vi "RS_FSP.vi"(4 "error in":T13, 7 "Command":string) -> (0 "error out":T13, 3 "Response":T11)   [LabVIEW 2018]
uses:
  MOKO_LabViewLibrary/MokoLowLevel/MokoLowLovelControl/MLLC_Error.ctl
  MOKO_LabViewLibrary/MokoLowLevel/MokoLowLovelControl/MLLC_Mode.ctl
  MOKO_LabViewLibrary/MokoLowLevel/MokoLowLovelControl/MLLC_Response.ctl
  MOKO_LabViewLibrary/MokoLowLevel/MokoLowLovelControl/MLLC_ConnectCluster.ctl
  MOKO_LabViewLibrary/MokoLowLevel/MokoLowLovelControl/MLLC_InterfaceType.ctl
  MOKO_LabViewLibrary/MokoLowLevel/MokoLowLovelControl/MLLC_OpenedSession.ctl
  MOKO_LabViewLibrary/MokoLowLevel/MokoLowLovelControl/MLLC_InterfaceSettings.ctl
  MOKO_LabViewLibrary/MokoLowLevel/MokoLowLovelControl/MLLC_InterfaceKind.ctl
  MOKO_LabViewLibrary/MokoLowLevel/MokoLowLovelControl/MLLC_DriverName.ctl
  MOKO_LabViewLibrary/MokoLowLevel/MokoLowLovelControl/MLLC_ErrorCode.ctl
  MOKO_LabViewLibrary/MokoLowLevel/MokoLowLovelControl/MLLC_ResponseInit.ctl
  MOKO_LabViewLibrary/MokoLowLevel/MokoLowLovelControl/MLLC_Request.ctl
  MOKO_LabViewLibrary/MokoLowLevel/MokoLowLovelControl/MLLC_Delay.ctl
panel:
  in  "Request":T1="*IDN?"
  in  "Response Init":T2="Rohde&Schwarz,FSP-30"
  in  "Error Code":T3=5450
  in  "Driver Name":T4="RS_FSP"
  in  "Settings":T10={"Saved Data"=variant, "Data"={"Connect"={"InterfaceType"=enum."VISA", "OpenedSession"="TCPIP0::169.254.1.110::inst0::INSTR", "InterfaceSettings"={"Interface"=enum."Ethernet", "EOS 4 read"=enum."LF (\\n)", "EOS 4 write"=enum."LF (\\n)", "TMO, ms"=10000, "Sett"=variant}}}}
  in  "Mode":T12=enum."Check"
  # "RS_FSP"
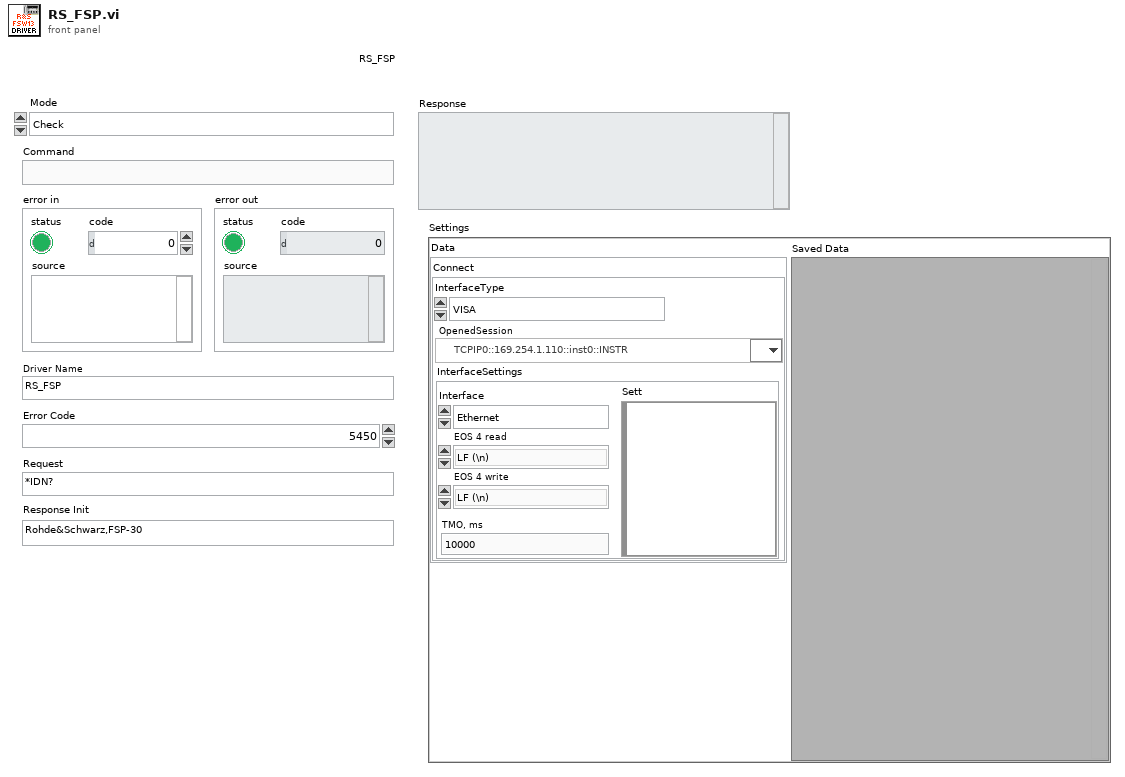
[diagram p1: front panel]
types:
  T1 = typedef "MLLC_Request.ctl" = string
  T2 = typedef "MLLC_ResponseInit.ctl" = string
  T3 = typedef "MLLC_ErrorCode.ctl" = u32
  T4 = typedef "MLLC_DriverName.ctl" = string
  T5 = typedef "MLLC_ConnectCluster.ctl" = cluster{"InterfaceType":T6, "OpenedSession":T7, "InterfaceSettings":T8}
  T6 = typedef "MLLC_InterfaceType.ctl" = enum16{"VISA", "Prologix USB-GPIB"}
  T7 = typedef "MLLC_OpenedSession.ctl" = refnum<visa-resource-name>
  T8 = typedef "MLLC_InterfaceSettings.ctl" = cluster{"Interface":T9, "EOS 4 read":enum16{"Default (=EOS 4 write)", "CR (\\r)", "LF (\\n)", "None"}, "EOS 4 write":enum16{"CR+LF (\\r\\n)", "CR (\\r)", "LF (\\n)", "None"}, "TMO, ms":i32, "Sett":variant}
  T9 = typedef "MLLC_InterfaceKind.ctl" = enum16{"RS232", "GPIB", "USB", "Ethernet", "another"}
  T10 = cluster{"Saved Data":variant, "Data":cluster{"Connect":T5}}
  T11 = typedef "MLLC_Response.ctl" = string
  T12 = typedef "MLLC_Mode.ctl" = enum16{"get", "set", "close", "Init", "Check"}
  T13 = typedef "MLLC_Error.ctl" = errorcluster
  T14 = typedef "MLLC_Delay.ctl" = dbl
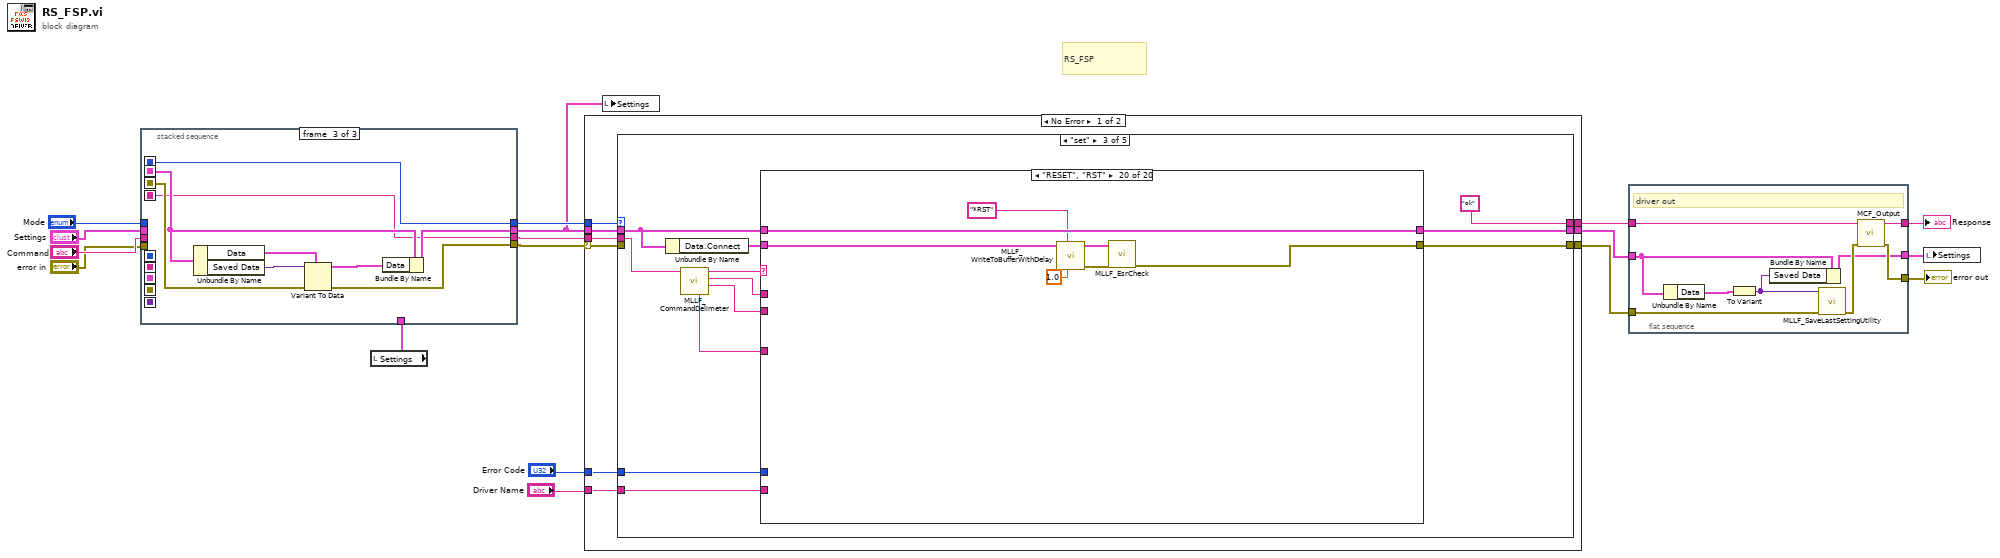
[diagram p0: block diagram]
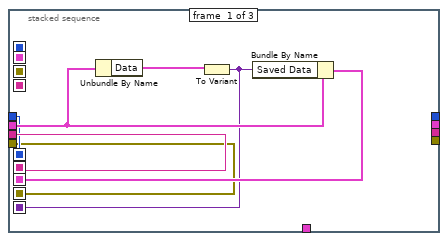
[diagram p2: hidden frame]
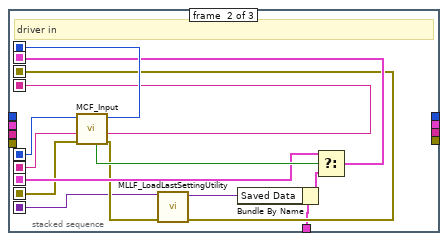
[diagram p3: hidden frame]
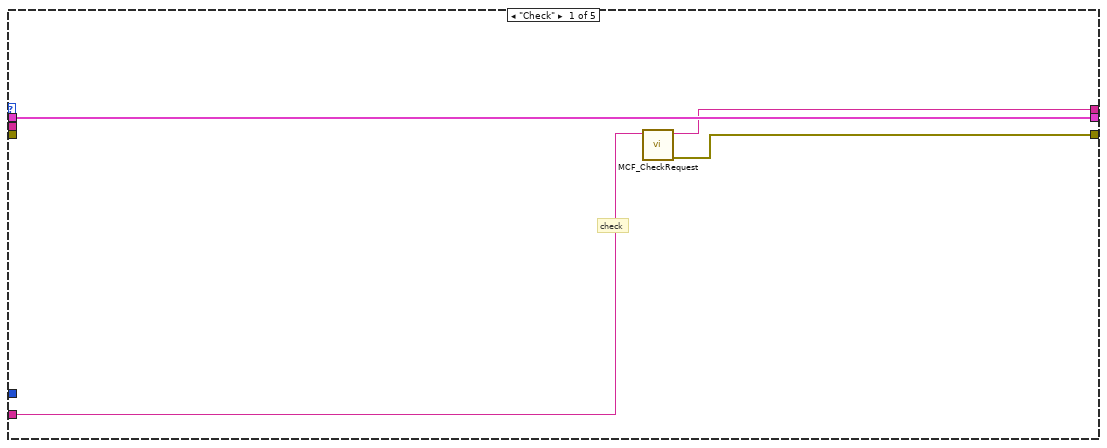
[diagram p4: hidden frame]
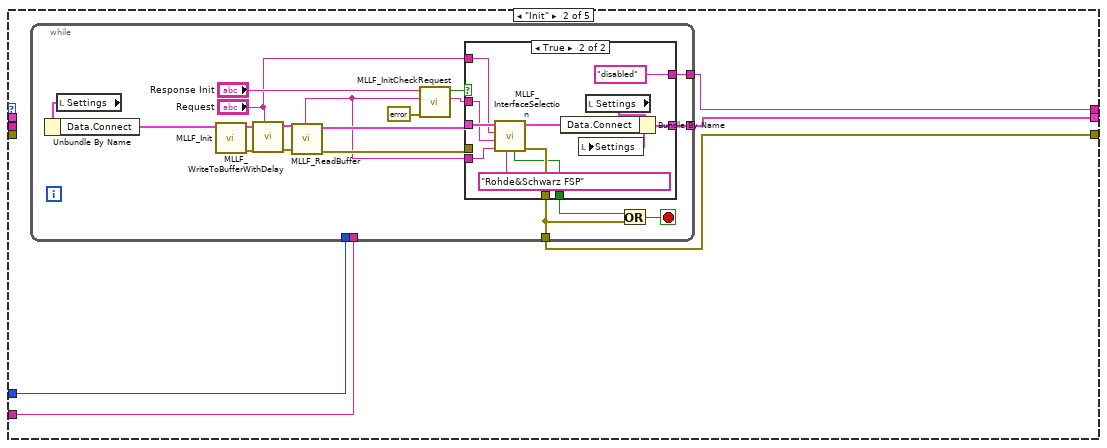
[diagram p5: hidden frame]
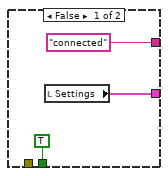
[diagram p6: hidden frame]
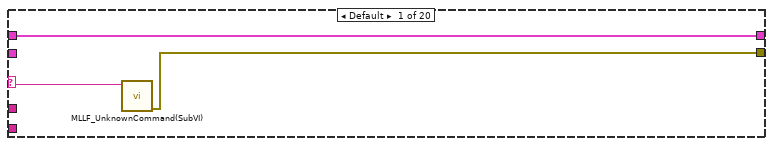
[diagram p7: hidden frame]
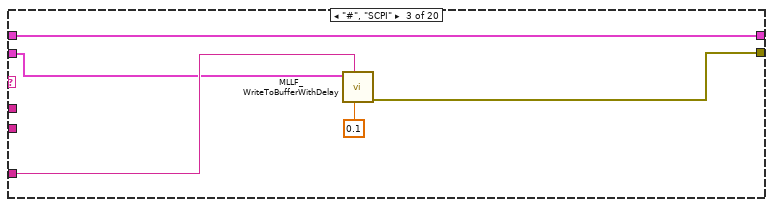
[diagram p9: hidden frame]
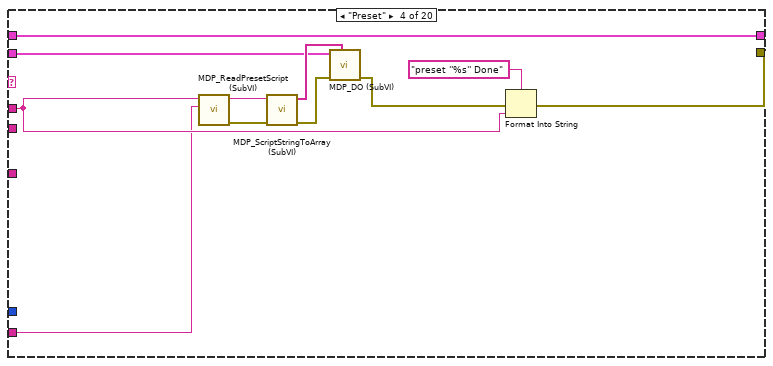
[diagram p10: hidden frame]
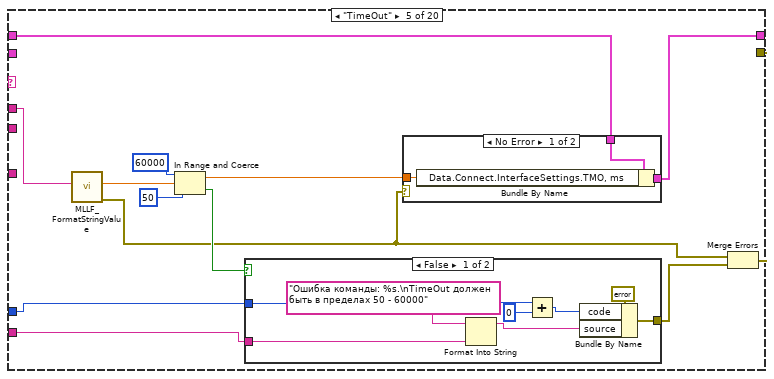
[diagram p11: hidden frame]
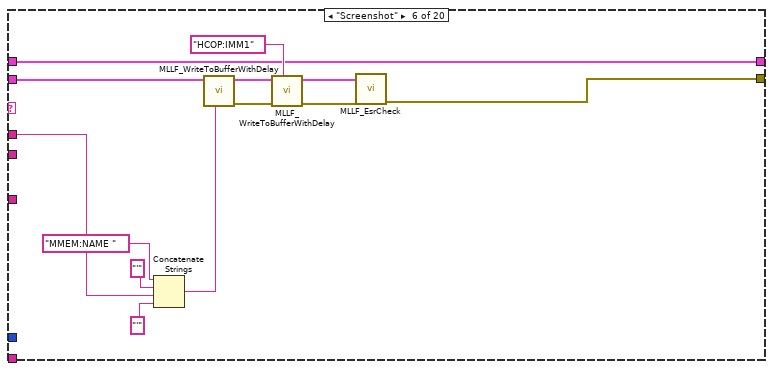
[diagram p14: hidden frame]
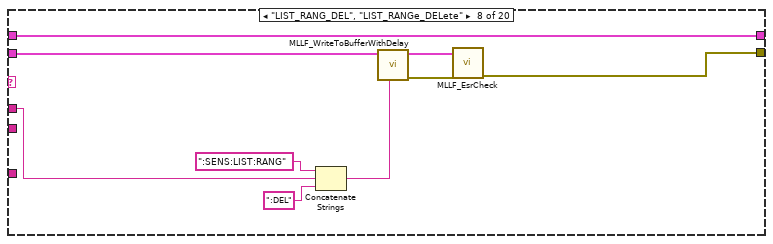
[diagram p16: hidden frame]
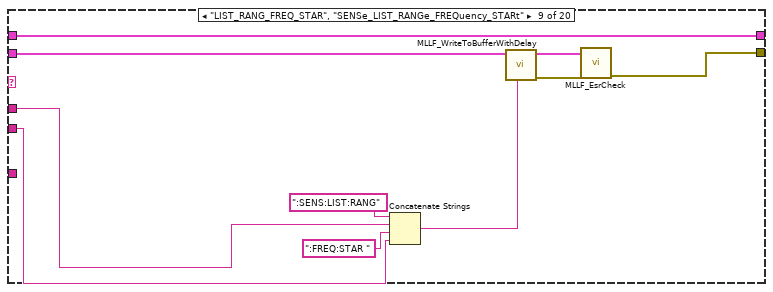
[diagram p17: hidden frame]
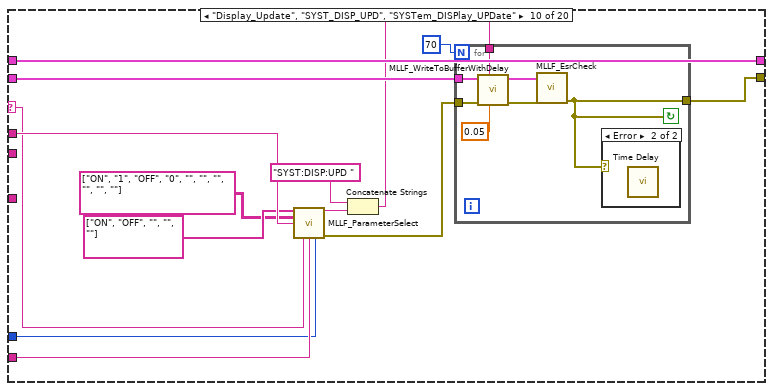
[diagram p18: hidden frame]
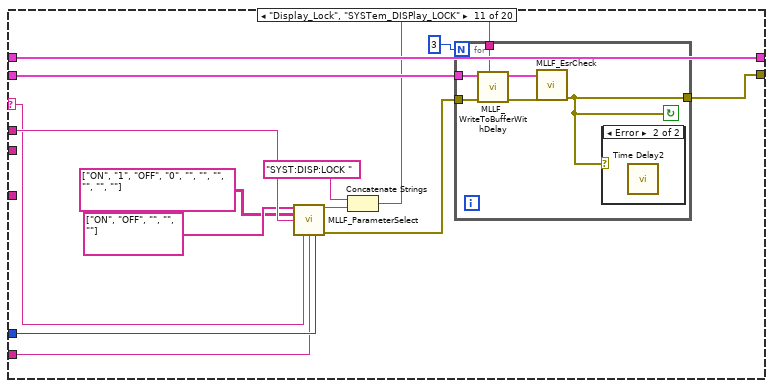
[diagram p20: hidden frame]
diagram:
  # "RS_FSP"
  n1 = local read "Settings"() -> (w15:T10)
  n2 = stacked-sequence {
    seq-local: [w20 _ _] -> [_ w36 _]
    seq-local: [w19 _ _] -> [_ w37 _]
    seq-local: [w22 _ _] -> [_ w32 _]
    seq-local: [w18 _ _] -> [_ w31 _]
    seq-local: [w21 _ _] -> [_ w27 _]
    seq-local: [_ w28 _] -> [_ _ w44]
    seq-local: [_ w38 _] -> [_ _ w41]
    seq-local: [_ w35 _] -> [_ _ w40]
    seq-local: [_ w34 _] -> [_ _ w45]
    tunnel: "Command" -> [w20 _ _]
    tunnel: "Mode" -> [w19 _ _]
    tunnel: "error in" -> [w18 _ _]
    tunnel: "Settings" -> [w23 _ _]
    tunnel: w15 -> [_ w26 _]
    tunnel: [_ _ w40] -> w8
    tunnel: [_ _ w43] -> w9
    tunnel: [_ _ w42] -> w7
    tunnel: [_ _ w41] -> w10
    frame #0 {
      n3 = Unbundle By Name(w23) -> ("Data"=w24:cluster{"Connect":T5})
      n4 = To Variant(anything=w24) -> (Variant=w21:variant)
      n5 = Bundle By Name(cluster=w23, "Saved Data"=w21) -> (w22:T10)
    }
    frame #1 {
      # "driver in"
      n6 = call "MCF_Input.vi"("Error In"=w31, "Command in"=w36, "Mode in"=w37) -> ("Error Out"=w30:errorcluster, "Command out"=w35:string, "Mode out"=w38:T12, "Boolean"=w33:bool)  [unwired: 5 in]
      n7 = call "MLLF_LoadLastSettingUtility.vi"("Error In"=w30, "Save data in"=w27) -> ("Error Out"=w28:errorcluster, "Save data out"=w25:variant)  [unwired: 8 in]
      n8 = Bundle By Name(cluster=w26, "Saved Data"=w25) -> (w29:T10)
      n9 = Select(t=w32, s=w33, f=w29) -> (s? t:f=w34:T10)
    }
    frame #2 {
      n10 = Unbundle By Name(w45) -> ("Data"=w46:cluster{"Connect":T5}, "Saved Data"=w39:variant)
      n11 = Variant To Data(error in=w44, type=w46, Variant=w39) -> (data=w47:cluster{"Connect":T5}, error out=w42:errorcluster)
      n12 = Bundle By Name(cluster=w45, "Data"=w47) -> (w43:T10)
    }
  }
  n13 = case shown="No Error" w7 {
    selector: w7 -> [w52 w426]
    tunnel: [w54 w426] -> w4
    tunnel: w10 -> [w56 _]
    tunnel: [w55 "error" ("Output String")] -> w6
    tunnel: w8 -> [w53 _]
    tunnel: w9 -> [w49 w425]
    tunnel: "Error Code" -> [w51 _]
    tunnel: "Driver Name" -> [w50 _]
    tunnel: [w48 w425] -> w5
    frame No Error {
      n14 = case shown="\"set\"" w56 {
        tunnel: [w58 w63 "ok" ("Output String") w342 "close" ("Output String")] -> w55
        tunnel: [w57 w62 w103 w345 w422] -> w54
        tunnel: w53 -> [_ _ w110 w351 _]
        tunnel: w52 -> [_ _ _ _ _]
        tunnel: w51 -> [_ w65 w109 w348 _]
        tunnel: w50 -> [w59 w64 w106 w347 _]
        tunnel: w49 -> [w60 _ w108 w350 w421]
        tunnel: [w60 w61 w107 w349 w421] -> w48
        frame "Check" {
          # "check"
          # "Проверка подленности пользователя в соответствии с протоколом MD5."
          n15 = call "MCF_CheckRequest.vi"("Driver Name"=w59) -> ("Error Out"=w57:errorcluster, "Output String"=w58:string)  [unwired: 9 in]
        }
        frame "Init" {
          # "Тут проходит инициализация оборудования"
          n16 = while {
            tunnel: [w78] -> w62
            tunnel: w65 -> [_]
            tunnel: w64 -> [_]
            tunnel: [w75] -> w63
            tunnel: [w76] -> w61
            stop <- w77 stop-if-true
            n17 = local read "Settings"() -> (w80:T10)
            n18 = Unbundle By Name(w80) -> ("Data.Connect"=w73:T5)
            n19 = call "MLLF_Init.vi"("DriverConnect in"=w73) -> ("Error Out"=w82:errorcluster, "DriverConnect out"=w81:T5)  [unwired: 7 in]
            n20 = call "MLLF_WriteToBufferWithDelay.vi"("Command"="Request", "Error In"=w82, "DriverConnect in"=w81) -> ("Error Out"=w84:errorcluster, "DriverConnect out"=w83:T5)  [unwired: 7 in]
            n21 = call "MLLF_ReadBuffer.vi"("Error In"=w84, "DriverConnect in"=w83) -> ("Error Out"=w68:errorcluster, "DriverConnect out"=w69:T5, "String"=w66:string)  [unwired: 6 in]
            n22 = call "MLLF_InitCheckRequest.vi"("error in (no error)"=errorcluster {"status"=FALSE, "code"=0, "source"=""}, "Answer"=w66, "Response Init"="Response Init") -> ("ResponseInit out"=w71:string, "Design"=w72:bool)  [unwired: 5 in, 2 out]
            n23 = case shown="True" w72 {
              tunnel: w69 -> [_ w97]
              tunnel: [TRUE w91] -> w79
              tunnel: [_ w98] -> w78
              tunnel: [w86 w93] -> w76
              tunnel: ["connected" "disabled"] -> w75
              tunnel: w68 -> [_ _]
              tunnel: w71 -> [_ w90]
              tunnel: "Request" -> [_ w89]
              tunnel: w66 -> [_ w88]
              frame False {
                n24 = local read "Settings"() -> (w86:T10)
              }
              frame True {
                n25 = call "MLLF_InterfaceSelection.vi"("Driver Name"="Rohde&Schwarz FSP" ("String"), "Answer:"=w88, "Response"=w90, "Request"=w89, "DriverConnect in"=w97) -> ("error out"=w98:T13, "DriverConnect out"=w95:T5, "stop init?"=w91:bool)  [unwired: 2 in, 2 out]
                n26 = local read "Settings"() -> (w94:T10)
                n27 = Bundle By Name(cluster=w94, "Data.Connect"=w95) -> (w93:T10)
                n28 = local write "Settings"(w93) -> ()
              }
            }
            n29 = Or(x=w79, y=w78) -> (x .or. y?=w77:bool)
          }
        }
        frame "set" {
          # "Тут реализованы функции DriverSet"
          n30 = Unbundle By Name(w108) -> ("Data.Connect"=w104:T5)
          n31 = call "MLLF_CommandDelimeter.vi"("command with param"=w110) -> ("param 2"=w100:string, "param 1"=w101:string, "command"=w102:string, "Spit delimetre"=w99:string)  [unwired: 6 in, 1 out]
          n32 = case shown="\"RESET\", \"RST\"" w102 {
            selector: w102 -> [w112 _ _ _ _ _ _ _ _ w189 w210 w230 w250 w270 _ _ _ _ _ _]
            tunnel: w108 -> [w113 w114 w119 w120 w133 w160 w169 w177 w187 w202 w223 w243 w263 w283 w294 w304 w318 w327 w333 w340]
            tunnel: [w113 w114 w119 w120 w132 w160 w169 w177 w187 w202 w223 w243 w263 w283 w294 w304 w318 w327 w333 w340] -> w107
            tunnel: w101 -> [_ _ _ w123 w131 w159 _ w171 w180 w199 w220 w240 w260 w280 _ _ w311 _ _ _]
            tunnel: w109 -> [_ _ _ _ w135 _ _ _ _ w190 w212 w232 w251 w272 _ _ _ _ _ _]
            tunnel: w106 -> [_ _ _ w122 w136 _ _ _ _ w191 w211 w231 w252 w271 _ _ _ _ _ _]
            tunnel: [w111 _ w117 w121 w134 w156 _ w176 w186 w201 w222 w242 w262 w282 w293 w303 w317 w326 w332 w339] -> w103
            tunnel: w104 -> [_ _ w115 w124 _ w168 _ w178 w188 w200 w221 w241 w261 w281 w292 w302 w316 w325 w331 w338]
            tunnel: w100 -> [_ _ _ _ _ _ _ _ w179 _ _ _ _ _ _ _ w310 _ _ _]
            tunnel: w99 -> [_ _ w116 _ _ _ _ _ _ _ _ _ _ _ _ _ _ _ _ _]
            frame Default {
              n33 = call "MLLF_UnknownCommand(SubVI).vi"("Unknown command"=w112) -> ("error out"=w111:errorcluster)  [unwired: 10 in]
            }
            frame "______________ Standart ________________" {
            }
            frame "#", "SCPI" {
              n34 = call "MLLF_WriteToBufferWithDelay.vi"("Delay Time ( 0,05 s)"=0.1 ("Delay Time (s)"), "Command"=w116, "DriverConnect in"=w115) -> ("Error Out"=w117:errorcluster)  [unwired: 7 in, 1 out]
            }
            frame "Preset" {
              n35 = call "MDP_ReadPresetScript (SubVI).vi"("Driver Name"=w122, "String in"=w123) -> ("Error Out"=w128:errorcluster, "String out"=w129:string)  [unwired: 8 in]
              n36 = call "MDP_ScriptStringToArray (SubVI).vi"("Error In"=w128, "String script"=w129) -> ("Error Out"=w130:errorcluster, "Array script"=w125:string[])  [unwired: 8 in]
              n37 = call "MDP_DO (SubVI).vi"("Array script"=w125, "Error in (no error)"=w130, "DriverConnect in"=w124) -> ("Error Out"=w126:errorcluster)  [unwired: 7 in, 1 out]
              n38 = Format Into String(format string="preset ''%s'' Done" ("Befor substring"), error in=w126, w123) -> (error out=w121:errorcluster)  [unwired: 1 in, 1 out]
            }
            frame "TimeOut" {
              n39 = call "MLLF_FormatStringValue.vi"("String Value"=w131) -> ("error out"=w138:T13, "number"=w137:dbl)  [unwired: 8 in, 1 out]
              n40 = In Range and Coerce(upper limit=60000, x=w137, lower limit=50) -> (coerced(x)=w141:dbl, In Range?=w139:bool)
              n41 = case shown="False" w139 {
                tunnel: [w150 _] -> w140
                tunnel: w135 -> [w149 _]
                tunnel: w136 -> [w148 _]
                frame False {
                  n42 = Format Into String(format string="Ошибка команды: %s.\nTimeOut должен быть в пределах 50 - 60000", w148) -> (resulting string=w152:string)  [unwired: 2 in, 1 out]
                  n43 = Add(x=w149, y=0) -> (x+y=w153:T3)
                  n44 = Bundle By Name(cluster=errorcluster {"status"=TRUE, "code"=0, "source"=""} ("error out"), "code"=w153, "source"=w152) -> (w150:errorcluster)
                }
                frame True {
                }
              }
              n45 = case shown="No Error" w138 {
                tunnel: [w146 w147] -> w132
                tunnel: w133 -> [w145 w147]
                tunnel: w141 -> [w144 _]
                frame No Error {
                  n46 = Bundle By Name(cluster=w145, "Data.Connect.InterfaceSettings.TMO, ms"=w144) -> (w146:T10)
                }
                frame Error {
                }
              }
              n47 = Merge Errors(w138, w140) -> (w134:errorcluster)
            }
            frame "Screenshot" {
              n48 = Concatenate Strings("MMEM:NAME " ("String"), "'" ("string"), w159, "'" ("string")) -> (w163:string)
              n49 = call "MLLF_WriteToBufferWithDelay.vi"("Command"=w163, "DriverConnect in"=w168) -> ("Error Out"=w162:errorcluster, "DriverConnect out"=w167:T5)  [unwired: 8 in]
              n50 = call "MLLF_WriteToBufferWithDelay.vi"("Command"="HCOP:IMM1" ("String"), "Error In"=w162, "DriverConnect in"=w167) -> ("Error Out"=w158:errorcluster, "DriverConnect out"=w157:T5)  [unwired: 7 in]
              n51 = call "MLLF_EsrCheck.vi"("error in"=w158, "DriverConnect in"=w157) -> ("error out"=w156:T13)  [unwired: 8 in, 1 out]
            }
            frame "________________________________________" {
            }
            frame "LIST_RANG_DEL", "LIST_RANGe_DELete" {
              n52 = Concatenate Strings(":SENS:LIST:RANG" ("String"), w171, ":DEL" ("string")) -> (w170:string)
              n53 = call "MLLF_WriteToBufferWithDelay.vi"("Command"=w170, "DriverConnect in"=w178) -> ("Error Out"=w174:errorcluster, "DriverConnect out"=w175:T5)  [unwired: 8 in]
              n54 = call "MLLF_EsrCheck.vi"("error in"=w174, "DriverConnect in"=w175) -> ("error out"=w176:T13)  [unwired: 8 in, 1 out]
            }
            frame "LIST_RANG_FREQ_STAR", "SENSe_LIST_RANGe_FREQuency_STARt" {
              n55 = Concatenate Strings(":SENS:LIST:RANG" ("String"), w180, ":FREQ:STAR " ("string"), w179) -> (w181:string)
              n56 = call "MLLF_WriteToBufferWithDelay.vi"("Command"=w181, "DriverConnect in"=w188) -> ("Error Out"=w184:errorcluster, "DriverConnect out"=w185:T5)  [unwired: 8 in]
              n57 = call "MLLF_EsrCheck.vi"("error in"=w184, "DriverConnect in"=w185) -> ("error out"=w186:T13)  [unwired: 8 in, 1 out]
            }
            frame "Display_Update", "SYST_DISP_UPD", "SYSTem_DISPlay_UPDate" {
              n58 = call "MLLF_ParameterSelect.vi"("Command to equipment"=string[] ["ON", "OFF", "", "", ""], "Names"=string[][] [["ON", "1"], ["OFF", "0"], ["", ""], ["", ""], ["", ""]], "Input"=w199, "Command"=w189, "Driver Name"=w191, "Error Code"=w190) -> ("Choice"=w195:string, "Error Out"=w192:errorcluster)  [unwired: 8 in]
              n59 = Concatenate Strings("SYST:DISP:UPD " ("string"), w195) -> (w194:string)
              n60 = for {
                N: 70 -> [_]
                tunnel: [w204] -> w201
                tunnel: w200 -> [w207]
                tunnel: w194 -> [w206]
                tunnel: w192 -> [w205]
                stop <- w204 continue-if-true
                n61 = call "MLLF_WriteToBufferWithDelay.vi"("Delay Time ( 0,05 s)"=T14 0.05, "Command"=w206, "Error In"=w205, "DriverConnect in"=w207) -> ("Error Out"=w209:errorcluster, "DriverConnect out"=w208:T5)  [unwired: 6 in]
                n62 = call "MLLF_EsrCheck.vi"("error in"=w209, "DriverConnect in"=w208) -> ("error out"=w204:T13)  [unwired: 8 in, 1 out]
                n63 = case shown="Error" w204 {
                  frame No Error {
                  }
                  frame Error {
                    n64 = call "Time Delay"() -> ()  [unwired: 11 in, 1 out]
                  }
                }
              }
            }
            frame "Display_Lock", "SYSTem_DISPlay_LOCK" {
              n65 = call "MLLF_ParameterSelect.vi"("Command to equipment"=string[] ["ON", "OFF", "", "", ""], "Names"=string[][] [["ON", "1"], ["OFF", "0"], ["", ""], ["", ""], ["", ""]], "Input"=w220, "Command"=w210, "Driver Name"=w211, "Error Code"=w212) -> ("Choice"=w216:string, "Error Out"=w213:errorcluster)  [unwired: 8 in]
              n66 = Concatenate Strings("SYST:DISP:LOCK " ("string"), w216) -> (w215:string)
              n67 = for {
                N: 3 -> [_]
                tunnel: [w224] -> w222
                tunnel: w221 -> [w227]
                tunnel: w215 -> [w226]
                tunnel: w213 -> [w225]
                stop <- w224 continue-if-true
                n68 = call "MLLF_WriteToBufferWithDelay.vi"("Command"=w226, "Error In"=w225, "DriverConnect in"=w227) -> ("Error Out"=w229:errorcluster, "DriverConnect out"=w228:T5)  [unwired: 7 in]
                n69 = call "MLLF_EsrCheck.vi"("error in"=w229, "DriverConnect in"=w228) -> ("error out"=w224:T13)  [unwired: 8 in, 1 out]
                n70 = case shown="Error" w224 {
                  frame No Error {
                  }
                  frame Error {
                    n71 = call "Time Delay2"() -> ()  [unwired: 11 in, 1 out]
                  }
                }
              }
            }
            frame "INIT_CONT", "INITiate_CONTinuous" {
              n72 = call "MLLF_ParameterSelect.vi"("Command to equipment"=string[] ["ON", "OFF", "", "", ""], "Names"=string[][] [["ON", "1"], ["OFF", "0"], ["", ""], ["", ""], ["", ""]], "Input"=w240, "Command"=w230, "Driver Name"=w231, "Error Code"=w232) -> ("Choice"=w236:string, "Error Out"=w233:errorcluster)  [unwired: 8 in]
              n73 = Concatenate Strings(":INIT:CONT " ("string"), w236) -> (w235:string)
              n74 = for {
                N: 3 -> [_]
                tunnel: [w244] -> w242
                tunnel: w241 -> [w247]
                tunnel: w235 -> [w246]
                tunnel: w233 -> [w245]
                stop <- w244 continue-if-true
                n75 = call "MLLF_WriteToBufferWithDelay.vi"("Command"=w246, "Error In"=w245, "DriverConnect in"=w247) -> ("Error Out"=w249:errorcluster, "DriverConnect out"=w248:T5)  [unwired: 7 in]
                n76 = call "MLLF_EsrCheck.vi"("error in"=w249, "DriverConnect in"=w248) -> ("error out"=w244:T13)  [unwired: 8 in, 1 out]
                n77 = case shown="Error" w244 {
                  frame No Error {
                  }
                  frame Error {
                    n78 = call "Time Delay3"() -> ()  [unwired: 11 in, 1 out]
                  }
                }
              }
            }
            frame "CALC_SGR_CONT", "CALCulate_SGRam_CONTinuous" {
              n79 = call "MLLF_ParameterSelect.vi"("Command to equipment"=string[] ["ON", "OFF", "", "", ""], "Names"=string[][] [["ON", "1"], ["OFF", "0"], ["", ""], ["", ""], ["", ""]], "Input"=w260, "Command"=w250, "Driver Name"=w252, "Error Code"=w251) -> ("Choice"=w256:string, "Error Out"=w253:errorcluster)  [unwired: 8 in]
              n80 = Concatenate Strings(":CALC:SGR:CONT " ("string"), w256) -> (w255:string)
              n81 = for {
                N: 3 -> [_]
                tunnel: [w264] -> w262
                tunnel: w261 -> [w267]
                tunnel: w255 -> [w266]
                tunnel: w253 -> [w265]
                stop <- w264 continue-if-true
                n82 = call "MLLF_WriteToBufferWithDelay.vi"("Command"=w266, "Error In"=w265, "DriverConnect in"=w267) -> ("Error Out"=w269:errorcluster, "DriverConnect out"=w268:T5)  [unwired: 7 in]
                n83 = call "MLLF_EsrCheck.vi"("error in"=w269, "DriverConnect in"=w268) -> ("error out"=w264:T13)  [unwired: 8 in, 1 out]
                n84 = case shown="Error" w264 {
                  frame No Error {
                  }
                  frame Error {
                    n85 = call "Time Delay4"() -> ()  [unwired: 11 in, 1 out]
                  }
                }
              }
            }
            frame "CALC_SPEC_CONT", "CALCulate_SPECtrogram_CONTinuous" {
              n86 = call "MLLF_ParameterSelect.vi"("Command to equipment"=string[] ["ON", "OFF", "", "", ""], "Names"=string[][] [["ON", "1"], ["OFF", "0"], ["", ""], ["", ""], ["", ""]], "Input"=w280, "Command"=w270, "Driver Name"=w271, "Error Code"=w272) -> ("Choice"=w276:string, "Error Out"=w273:errorcluster)  [unwired: 8 in]
              n87 = Concatenate Strings(":CALC:SPEC:CONT " ("string"), w276) -> (w275:string)
              n88 = for {
                N: 3 -> [_]
                tunnel: [w284] -> w282
                tunnel: w281 -> [w287]
                tunnel: w275 -> [w286]
                tunnel: w273 -> [w285]
                stop <- w284 continue-if-true
                n89 = call "MLLF_WriteToBufferWithDelay.vi"("Command"=w286, "Error In"=w285, "DriverConnect in"=w287) -> ("Error Out"=w289:errorcluster, "DriverConnect out"=w288:T5)  [unwired: 7 in]
                n90 = call "MLLF_EsrCheck.vi"("error in"=w289, "DriverConnect in"=w288) -> ("error out"=w284:T13)  [unwired: 8 in, 1 out]
                n91 = case shown="Error" w284 {
                  frame No Error {
                  }
                  frame Error {
                    n92 = call "Time Delay6"() -> ()  [unwired: 11 in, 1 out]
                  }
                }
              }
            }
            frame "CALC_SGR_CLE", "CALCulate_SGRam_CLEar" {
              n93 = for {
                N: 3 -> [_]
                tunnel: [w295] -> w293
                tunnel: w292 -> [w297]
                tunnel: "CALC:SGR:CLE" ("string") -> [w296]
                stop <- w295 continue-if-true
                n94 = call "MLLF_WriteToBufferWithDelay.vi"("Command"=w296, "DriverConnect in"=w297) -> ("Error Out"=w299:errorcluster, "DriverConnect out"=w298:T5)  [unwired: 8 in]
                n95 = call "MLLF_EsrCheck.vi"("error in"=w299, "DriverConnect in"=w298) -> ("error out"=w295:T13)  [unwired: 8 in, 1 out]
                n96 = case shown="Error" w295 {
                  frame No Error {
                  }
                  frame Error {
                    n97 = call "Time Delay7"() -> ()  [unwired: 11 in, 1 out]
                  }
                }
              }
            }
            frame "CALC_SPEC_CLE", "CALCulate_SPECtrogram_CLEar" {
              n98 = for {
                N: 3 -> [_]
                tunnel: [w305] -> w303
                tunnel: w302 -> [w307]
                tunnel: "CALC:SPEC:CLE" ("string") -> [w306]
                stop <- w305 continue-if-true
                n99 = call "MLLF_WriteToBufferWithDelay.vi"("Command"=w306, "DriverConnect in"=w307) -> ("Error Out"=w309:errorcluster, "DriverConnect out"=w308:T5)  [unwired: 8 in]
                n100 = call "MLLF_EsrCheck.vi"("error in"=w309, "DriverConnect in"=w308) -> ("error out"=w305:T13)  [unwired: 8 in, 1 out]
                n101 = case shown="Error" w305 {
                  frame No Error {
                  }
                  frame Error {
                    n102 = call "Time Delay8"() -> ()  [unwired: 11 in, 1 out]
                  }
                }
              }
            }
            frame "INIT_OPC", "INITiate_OPC" {
              n103 = case shown="\"Timeout\", \"TMO\"" w311 {
                tunnel: w310 -> [_ w321]
                tunnel: [20.0 w320] -> w312
                frame "False", Default {
                }
                frame "Timeout", "TMO" {
                  n104 = Scan From String(input string=w321) -> (output 1=w320:dbl)  [unwired: 4 in, 3 out]
                }
              }
              n105 = call "MLLF_WriteToBufferWithDelay.vi"("Delay Time ( 0,05 s)"=w312, "Command"="INIT:SPUR" ("string"), "DriverConnect in"=w316) -> ("Error Out"=w314:errorcluster, "DriverConnect out"=w313:T5)  [unwired: 7 in]
              n106 = call "MLLF_EsrCheck.vi"("error in"=w314, "DriverConnect in"=w313) -> ("error out"=w317:T13)  [unwired: 8 in, 1 out]
            }
            frame "ListXAdj" {
              # ":SENS:LIST:XADJ;*WAI"
              n107 = call "MLLF_WriteToBufferWithDelay.vi"("Command"=":SENS:LIST:XADJ" ("string"), "DriverConnect in"=w325) -> ("Error Out"=w323:errorcluster, "DriverConnect out"=w322:T5)  [unwired: 8 in]
              n108 = call "MLLF_EsrCheck.vi"("error in"=w323, "DriverConnect in"=w322) -> ("error out"=w326:T13)  [unwired: 8 in, 1 out]
            }
            frame "SensAdjAll" {
              # ":SENS:ADJ:ALL;*WAI"
              n109 = call "MLLF_WriteToBufferWithDelay.vi"("Command"=":SENS:ADJ:ALL;*WAI" ("string"), "DriverConnect in"=w331) -> ("Error Out"=w329:errorcluster, "DriverConnect out"=w328:T5)  [unwired: 8 in]
              n110 = call "MLLF_EsrCheck.vi"("error in"=w329, "DriverConnect in"=w328) -> ("error out"=w332:T13)  [unwired: 8 in, 1 out]
            }
            frame "RESET", "RST" {
              n111 = call "MLLF_WriteToBufferWithDelay.vi"("Delay Time ( 0,05 s)"=1.0, "Command"="*RST" ("string"), "DriverConnect in"=w338) -> ("Error Out"=w336:errorcluster, "DriverConnect out"=w335:T5)  [unwired: 7 in]
              n112 = call "MLLF_EsrCheck.vi"("error in"=w336, "DriverConnect in"=w335) -> ("error out"=w339:T13)  [unwired: 8 in, 1 out]
            }
          }
        }
        frame "get" {
          # "Тут реализованы функции DriverGet"
          n113 = Unbundle By Name(w350) -> ("Data.Connect"=w346:T5)
          n114 = call "MLLF_CommandDelimeter.vi"("command with param"=w351) -> ("param 1"=w343:string, "command"=w344:string, "Spit delimetre"=w341:string)  [unwired: 6 in, 2 out]
          n115 = case shown="\"TraceDataSpur\"" w344 {
            selector: w344 -> [w353 _ _ _ _ _ _ _ _]
            tunnel: [w352 _ w357 _ _ _ w382 w396 w405] -> w345
            tunnel: w348 -> [_ _ _ _ _ _ _ _ _]
            tunnel: [w354 w355 w366 w369 w370 w371 w381 w395 w419] -> w349
            tunnel: w350 -> [w354 w355 w366 w369 w370 w371 w381 w395 w419]
            tunnel: w346 -> [_ _ w359 _ _ _ w383 w397 w414]
            tunnel: w347 -> [_ _ _ _ _ _ _ _ w407]
            tunnel: [_ _ w356 w367 _ _ w374 w391 "write to Data.txt" ("output")] -> w342
            tunnel: w343 -> [_ _ _ _ _ _ _ _ _]
            tunnel: w341 -> [_ _ w358 _ _ _ _ _ _]
            frame Default {
              # "DEFAULT"
              n116 = call "MLLF_UnknownCommand(SubVI).vi"("Unknown command"=w353) -> ("error out"=w352:errorcluster)  [unwired: 10 in]
            }
            frame "______________ Standart ________________" {
            }
            frame "#", "SCPI" {
              n117 = call "MLLF_ClearBuffer.vi"("Timeout(default = 300 ms)"=u32 100 ("Timeout"), "DriverConnect in"=w359) -> ("Error Out"=w360:errorcluster, "DriverConnect out"=w361:T5)  [unwired: 6 in, 1 out]
              n118 = call "MLLF_WriteToBufferWithDelay.vi"("Delay Time ( 0,05 s)"=0.1 ("Delay Time (s)"), "Command"=w358, "Error In"=w360, "DriverConnect in"=w361) -> ("Error Out"=w364:errorcluster, "DriverConnect out"=w365:T5)  [unwired: 6 in]
              n119 = call "MLLF_ReadBuffer.vi"("Error In"=w364, "DriverConnect in"=w365) -> ("Error Out"=w357:errorcluster, "String"=w356:string)  [unwired: 6 in, 1 out]
            }
            frame "TIMEOUT" {
              # "Время ожидания ответа от прибора."
              n120 = Unbundle By Name(w369) -> ("Data.Connect.InterfaceSettings.TMO, ms"=w368:i32)
              n121 = Format Value(value (0)=w368) -> (output string=w367:string)  [unwired: 2 in]
            }
            frame "________________________________________" {
            }
            frame "------ID-------" {
            }
            frame "model" {
              n122 = call "RS_FSP_FASTQUERY.vi"("input"="*IDN?", "DriverConnect in"=w383) -> ("error out"=w382:T13, "output"=w380:string)  [unwired: 7 in, 1 out]
              n123 = for {
                N: 4 -> [_]
                shift-right: [w385] -> _
                shift-left: w380 -> [w388]
                tunnel: [w387] -> w379 mode=indexing
                stop <- w386 stop-if-true
                n124 = Match Pattern(string=w388, regular expression=",") -> (before substring=w387:string, after substring=w385:string)  [unwired: 1 in, 2 out]
                n125 = Empty String/Path?(string/path=w385) -> (empty?=w386:bool)
              }
              n126 = Index Array(array=w379, index #1=0 ("index"), index #2=1 ("index")) -> (element #1=w377:string, element #2=w375:string)
              n127 = Concatenate Strings(w377, " " ("string"), w375) -> (w374:string)
            }
            frame "FW", "ver", "version" {
              n128 = call "RS_FSP_FASTQUERY.vi"("input"="*IDN?", "DriverConnect in"=w397) -> ("error out"=w396:T13, "output"=w392:string)  [unwired: 7 in, 1 out]
              n129 = for {
                N: 4 -> [_]
                shift-right: [w399] -> _
                shift-left: w392 -> [w402]
                tunnel: [w401] -> w394 mode=indexing
                stop <- w400 stop-if-true
                n130 = Match Pattern(string=w402, regular expression=",") -> (before substring=w401:string, after substring=w399:string)  [unwired: 1 in, 2 out]
                n131 = Empty String/Path?(string/path=w399) -> (empty?=w400:bool)
              }
              n132 = Index Array(array=w394, index=3) -> (element=w391:string)
            }
            frame "TraceDataSpur" {
              # "TRAC:DATA? SPUR"
              n133 = call "MLLF_WriteToBuffer.vi"("String"="TRAC:DATA? SPUR", "DriverConnect in"=w414) -> ("error out"=w415:T13, "DriverConnect out"=w416:T5)  [unwired: 6 in]
              n134 = call "MLLF_ReadBuffer.vi"("Error In"=w415, "DriverConnect in"=w416) -> ("Error Out"=w412:errorcluster, "DriverConnect out"=w413:T5, "String"=w417:string)  [unwired: 6 in]
              n135 = call <vilib>:"Trim Whitespace.vi"("string"=w417) -> ("trimmed string"=w411:string)  [unwired: 1 in]
              n136 = call "MLLF_EsrCheck.vi"("error in"=w412, "DriverConnect in"=w413) -> ("error out"=w406:T13)  [unwired: 8 in, 1 out]
              n137 = call "RS_FSP_ConvIntoFormatString.vi"("Mode"=enum16{"Value", "Status"}."Value", "Error In"=w406, "input string"=w411) -> ("Error Out"=w409:errorcluster, "output"=w408:string)  [unwired: 7 in]
              n138 = call "RS_FSP_SAve to datafile (SubVI).vi"("Error In"=w409, "Driver Name"=w407, "output"=w408) -> ("error out"=w405:errorcluster)  [unwired: 8 in]
            }
          }
        }
        frame "close" {
          # "Завершение сессии"
          n139 = Unbundle By Name(w421) -> ("Data.Connect.OpenedSession"=w423:T7)
          n140 = VISA Close(VISA resource name=w423) -> (error out=w422:errorcluster)  [unwired: 1 in]
        }
      }
    }
    frame Error {
    }
  }
  n141 = local write "Settings"(w9) -> ()
  n142 = flat-sequence {
    tunnel: [w435] -> w3
    tunnel: [w434] -> w1
    tunnel: w6 -> [w433]
    tunnel: w4 -> [w432]
    tunnel: w5 -> [w428]
    tunnel: [w430] -> w2
    frame #0 {
      # "driver out"
      n143 = Unbundle By Name(w428) -> ("Data"=w427:cluster{"Connect":T5})
      n144 = To Variant(anything=w427) -> (Variant=w429:variant)
      n145 = Bundle By Name(cluster=w428, "Saved Data"=w429) -> (w430:T10)
      n146 = call "MLLF_SaveLastSettingUtility.vi"("error in"=w432, "Saved Data"=w429) -> ("error out"=w431:T13)  [unwired: 8 in, 1 out]
      n147 = call "MCF_Output.vi"("Error In"=w431, "Input"=w433) -> ("Error Out"=w434:errorcluster, "Output"=w435:string)  [unwired: 8 in]
    }
  }
  n148 = local write "Settings"(w2) -> ()
  "error out" <- w1
  "Response" <- w3
